vi "Max compressed size.vi"(8 "error in (no error)":errorcluster, 10 "source size (bytes)":i32, 11 "lvzstd in":refnum<class "lvzstd.lvclass">) -> (0 "error out":errorcluster, 2 "maximum compressed size (bytes)":i32, 3 "lvzstd out":refnum<class "lvzstd.lvclass">)   [LabVIEW 2020, in "lvzstd.lvlib" / "lvzstd.lvclass"]
uses:
  lvzstd.lvclass
  lvzstd.lvclass/lvzstd.ctl
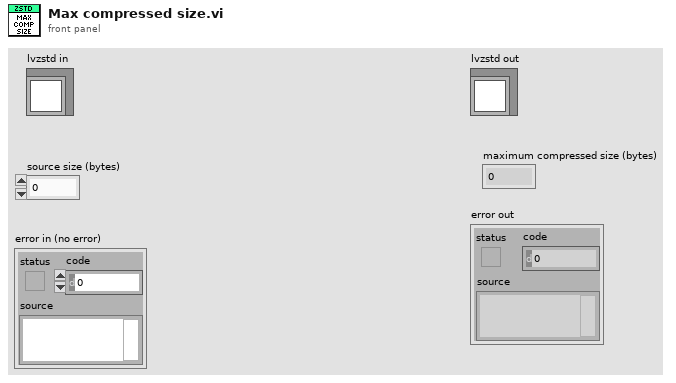
[diagram p1: front panel]
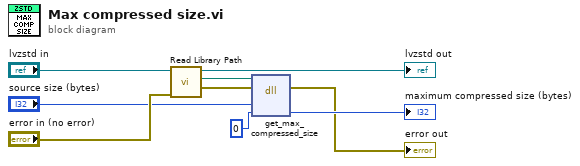
[diagram p0: block diagram]
diagram:
  n1 = call "Read Library Path.vi"("error in (no error)"="error in (no error)", "lvzstd in"="lvzstd in") -> ("error out"=w6:errorcluster, "Library Path"=w7:path, "lvzstd out"=→"lvzstd out":refnum<class "lvzstd.lvclass">)  [unwired: 7 in]
  n2 = dll-call lib="?" fn="get_max_compressed_size"(path in=w7, error in=w6, "source_size"="source size (bytes)", "max_compressed_size"=0) -> (error out=→"error out":errorcluster, "max_compressed_size"=→"maximum compressed size (bytes)":i32)  [unwired: 3 in, 1 out]
